vi "DEMO_05_Close_Open_BFUZAI.vi"() -> ()   [LabVIEW 2014]
uses:
  <vilib>/Instr/_visa.llb/VISA Configure Serial Port (Instr).vi
panel:
  in  "打开串口":bool
  in  "上位机控制":bool
  in  "读取标定":bool
  out "输出负载":dbl
  in  "负载数值":dbl
  in  "标定负载":bool
  in  "波特率":u32(ring)=9600 items=["75"=75, "110"=110, "134"=134, "150"=150, "300"=300, "600"=600, "1200"=1200, "1800"=1800, "2400"=2400, "4800"=4800, "7200"=7200, "9600"=9600, "14400"=14400, "19200"=19200, "28800"=28800, "38400"=38400, "56000"=56000, "57600"=57600, "115200"=115200, "128000"=128000, "230400"=230400]
  in  "奇偶":enum16{"None", "Odd", "Even", "Mark", "Space"}(ring) caption="校验"
  in  "VISA资源名称":refnum<visa-resource-name>="COM1"
  in  "通道选择":u16(ring) items=["一路", "二路", "三路"]
  # "标定负载以及读取负载"
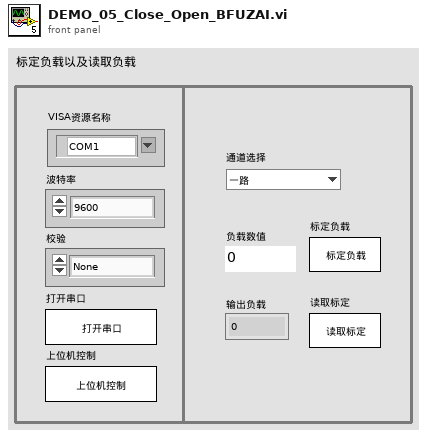
[diagram p1: front panel]
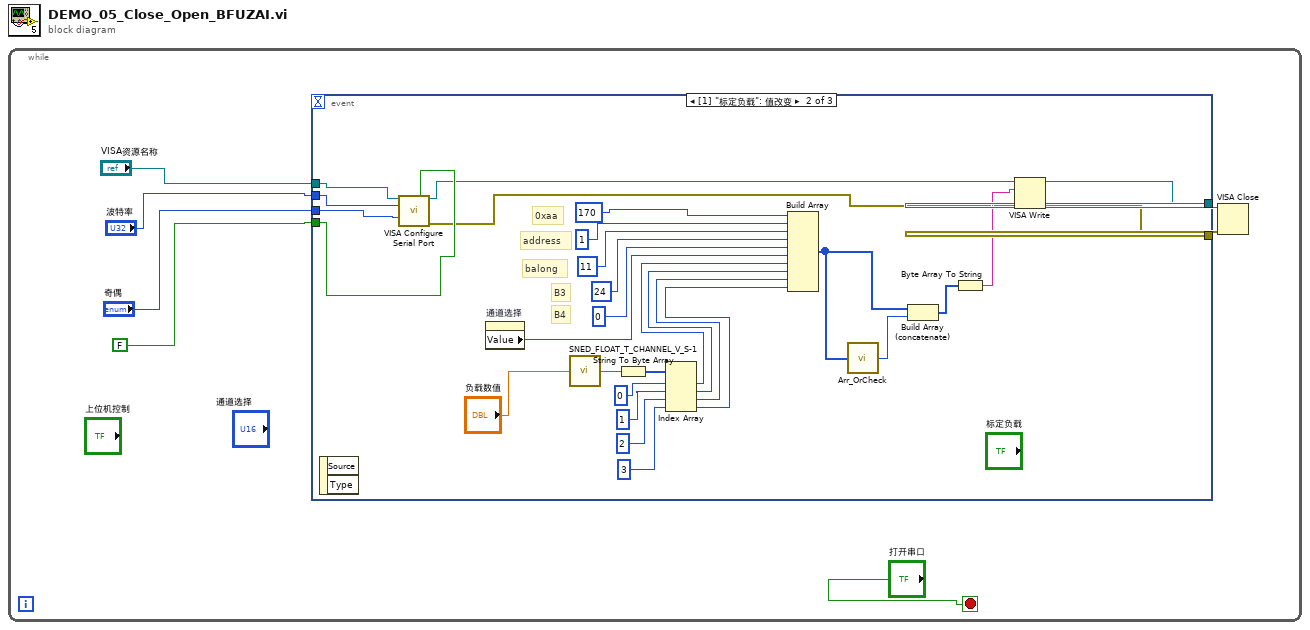
[diagram p0: block diagram]
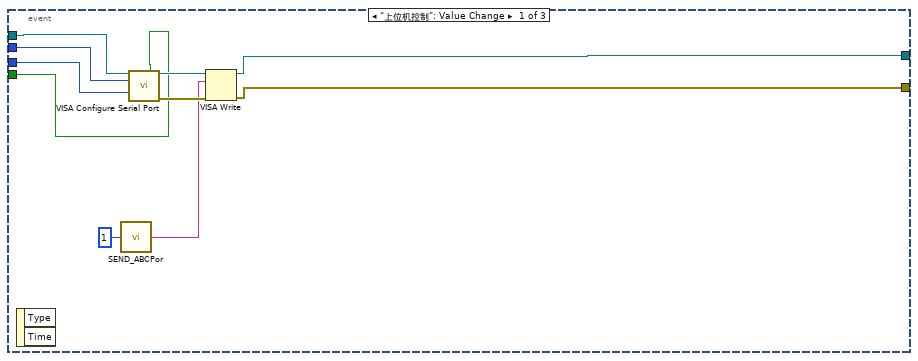
[diagram p2: hidden frame]
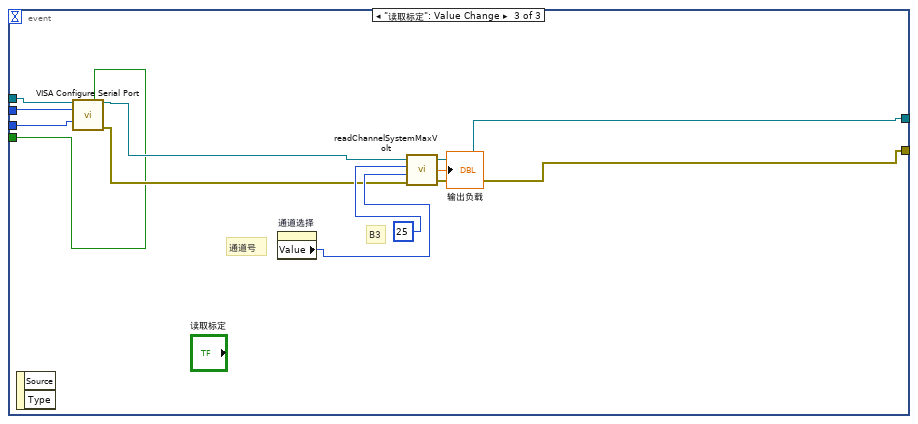
[diagram p3: hidden frame]
diagram:
  n1 = while {
    stop <- "打开串口" stop-if-true
    n2 = event shown="[1] \"标定负载\": 值改变" {
      selector: _ -> [_ _ _]
      dyn-events: _ -> [_ _ _]
      timeout: _ -> [_ _ _]
      tunnel: [w17 w19 w48] -> w6
      tunnel: [w16 w18 w49] -> w5
      tunnel: FALSE -> [w10 w46 w53]
      tunnel: "VISA资源名称" -> [w13 w44 w52]
      tunnel: "波特率" -> [w12 w43 w51]
      tunnel: "奇偶" -> [w11 w45 w50]
      event "上位机控制": Value Change {
        n3 = event-data() -> ()  [unwired: 1 in, 2 out]
        n4 = call "SEND_ABCPor.vi"("设备地址 1 开始"=1) -> ("输出字符串"=w8:string)
        n5 = call-poly "VISA Configure Serial Port"("VISA resource name"=w13, "Enable Termination\nChar (T)"=w10, "baud rate (9600)"=w12, "parity (0:none)"=w11) -> ("VISA resource name out"=w15:refnum<visa-resource-name>, "error out"=w14:errorcluster)  [unwired: 10 in]
        n6 = VISA Write(VISA resource name=w15, write buffer=w8, error in (no error)=w14) -> (VISA resource name out=w16:refnum<visa-resource-name>, error out=w17:errorcluster)  [unwired: 1 out]
      }
      event "标定负载": Value Change {
        # "B4"
        # "B3"
        # "balong"
        # "address"
        # "0xaa"
        n7 = event-data() -> ()  [unwired: 1 in, 2 out]
        n8 = call-poly "VISA Configure Serial Port"("VISA resource name"=w44, "Enable Termination\nChar (T)"=w46, "baud rate (9600)"=w43, "parity (0:none)"=w45) -> ("VISA resource name out"=w21:refnum<visa-resource-name>, "error out"=w20:errorcluster)  [unwired: 10 in]
        n9 = property on="通道选择" class="Ring (严格)"() -> ("Value"=w34:u16)  [unwired: 2 in, 2 out]
        n10 = call "SNED_FLOAT_T_CHANNEL_V_S-1.vi"("数据"="负载数值") -> ("字符串"=w42:string)
        n11 = String To Byte Array(string=w42) -> (unsigned byte array=w41:u8[])
        n12 = Index Array(array=w41, index #1=0, index #2=1, index #3=2, index #4=3) -> (element #1=w29:u8, element #2=w28:u8, element #3=w27:u8, element #4=w26:u8)
        n13 = Build Array(170, 1, 11, 24, 0, w34, w29, w28, w27, w26) -> (w25:i32[])
        n14 = call "Arr_OrCheck.vi"("数组"=w25) -> ("抑或的数据值"=w24:u8)
        n15 = Build Array (concatenate)(w25, w24) -> (w23:i32[])
        n16 = Byte Array To String(unsigned byte array=w23) -> (string=w22:string)
        n17 = VISA Write(VISA resource name=w21, write buffer=w22, error in (no error)=w20) -> (VISA resource name out=w18:refnum<visa-resource-name>, error out=w19:errorcluster)  [unwired: 1 out]
      }
      event "读取标定": Value Change {
        # "通道号"
        # "B3"
        n18 = event-data() -> ()  [unwired: 1 in, 2 out]
        n19 = call-poly "VISA Configure Serial Port"("VISA resource name"=w52, "Enable Termination\nChar (T)"=w53, "baud rate (9600)"=w51, "parity (0:none)"=w50) -> ("VISA resource name out"=w54:refnum<visa-resource-name>, "error out"=w55:errorcluster)  [unwired: 10 in]
        n20 = property on="通道选择" class="Ring (严格)"() -> ("Value"=w56:u16)  [unwired: 2 in, 2 out]
        n21 = call "readChannelSystemMaxVolt.vi"("error out 2"=w55, "通道号"=w56, "B3"=25, "VISA resource name out 2"=w54) -> ("error out"=w48:errorcluster, "输出变量"=→"输出负载":dbl, "VISA resource name out"=w49:refnum<visa-resource-name>)
      }
    }
    n22 = VISA Close(VISA resource name=w5, error in (no error)=w6) -> ()  [unwired: 1 out]
  }
